vi "Simple Add.vi"() -> ()   [LabVIEW 2017]
panel:
  out "x+y 2":dbl
  out "x+y":dbl
  in  "x":dbl
  in  "y":dbl
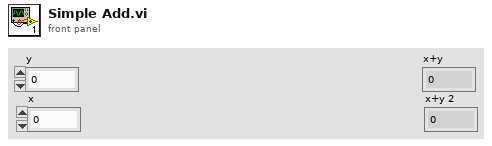
[diagram p1: front panel]
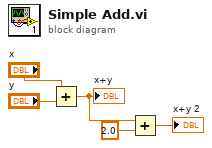
[diagram p0: block diagram]
diagram:
  n1 = Add(x="x", y="y") -> (x+y=w3:dbl)
  "x+y" <- w3
  n2 = Add(x=w3, y=2.0) -> (x+y=→"x+y 2":dbl)
